vi "Read Guidance Cluster.vi"(8 "error in (no error)":errorcluster, 11 "Supervisor in":refnum<class "Supervisor.lvclass">) -> (0 "error out":errorcluster, 2 "Guidance Cluster":T1, 3 "Supervisor out":refnum<class "Supervisor.lvclass">)   [LabVIEW 2012, in "Supervisor.lvclass"]
uses:
  Supervisor.lvclass
  Supervisor.lvclass/Supervisor.ctl
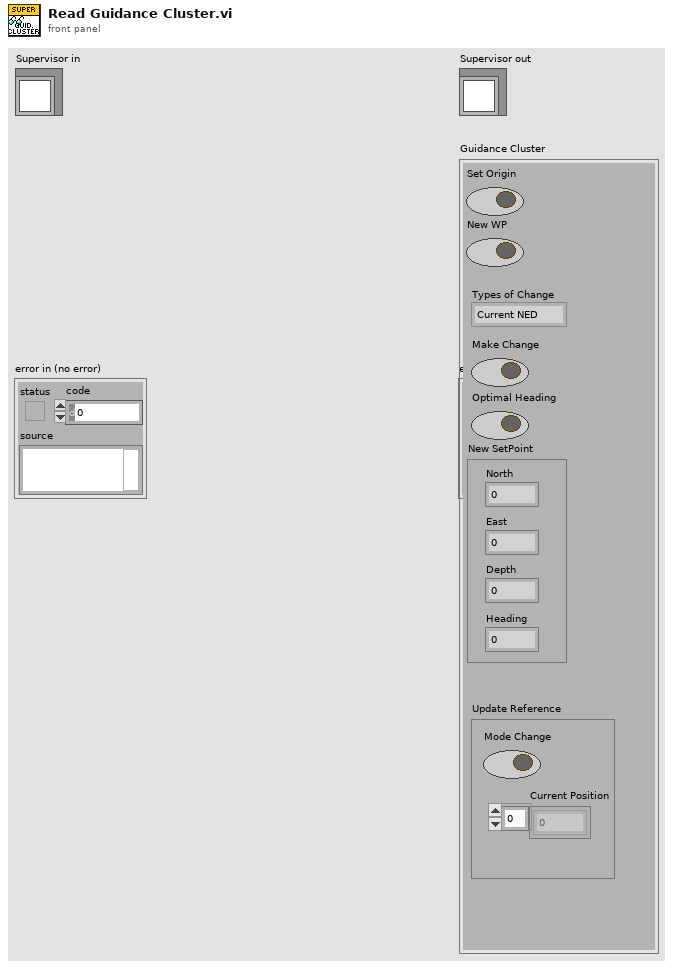
[diagram p1: front panel]
types:
  T1 = cluster{"Set Origin":bool, "New WP":bool, "Types of Change":enum16{"Current NED", "Change NED"}, "Make Change":bool, "Optimal Heading":bool, "New SetPoint":cluster{"North":dbl, "East":dbl, "Depth":dbl, "Heading":dbl}, "Update Reference":cluster{"Mode Change":bool, "Current Position":dbl[]}}
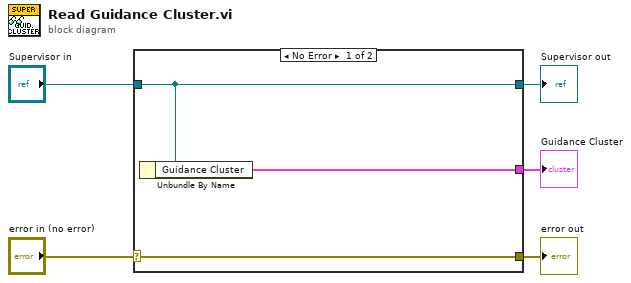
[diagram p0: block diagram]
diagram:
  n1 = case shown="No Error" "error in (no error)" {
    selector: "error in (no error)" -> [w8 w9]
    tunnel: [w8 w9] -> w4
    tunnel: [w7 w10] -> w2
    tunnel: "Supervisor in" -> [w7 w10]
    tunnel: [w6 _] -> w1
    frame No Error {
      n2 = Unbundle By Name(w7) -> ("Guidance Cluster"=w6:T1)
    }
    frame Error {
    }
  }
  "error out" <- w4
  "Supervisor out" <- w2
  "Guidance Cluster" <- w1
